vi "Dequeue Message.vi"(8 "error in (no error)":errorcluster, 10 "timeout in ms (-1)":i32=-1, 11 "Listening Queue":refnum<queue>) -> (0 "error out":errorcluster, 1 "Data":variant, 2 "Command":string, 3 "queue out":refnum<queue>, 4 "Time Stamp":timestamp, 5 "Destination":string, 7 "Source":string)   [LabVIEW 2018, in "Dynamic Reentrant.lvlib"]
uses:
  <userlib>/Dynamic Reentrant/Dynamic Reentrant.lvlib
  <userlib>/Dynamic Reentrant/Type Defs/Message.ctl
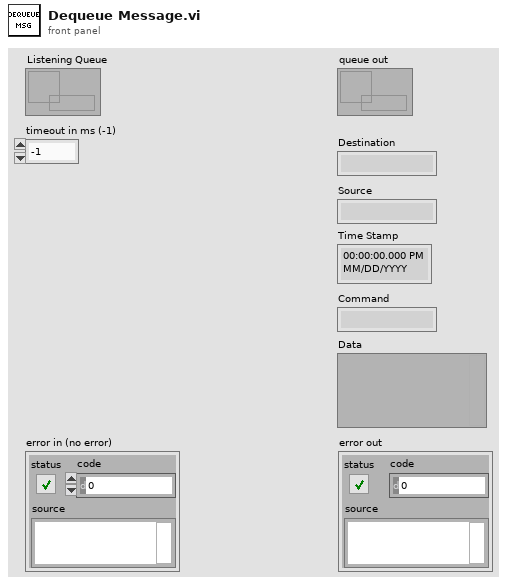
[diagram p1: front panel]
types:
  T1 = typedef "Dynamic Reentrant.lvlib/Message.ctl" = cluster{"Source":string, "Destination":string, "Time Stamp":timestamp, "Command":string, "Data":variant}
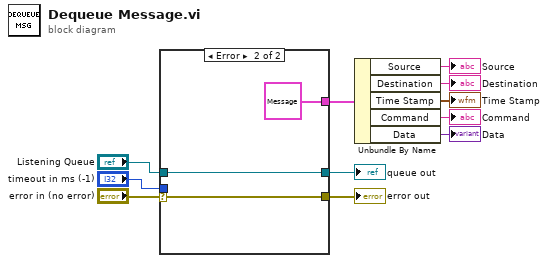
[diagram p0: block diagram]
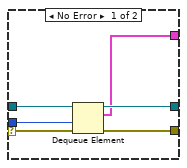
[diagram p2: hidden frame]
diagram:
  n1 = case shown="Error" "error in (no error)" {
    selector: "error in (no error)" -> [w12 w19]
    tunnel: "Listening Queue" -> [w17 w20]
    tunnel: "timeout in ms (-1)" -> [w16 _]
    tunnel: [w15 w19] -> w9
    tunnel: [w14 w20] -> w8
    tunnel: [w13 T1 {"Source"="", "Destination"="", "Time Stamp"=timestamp(0 s since 1904-01-01), "Command"="", "Data"=variant}] -> w7
    frame No Error {
      n2 = Dequeue Element(queue=w17, timeout in ms (-1)=w16, error in (no error)=w12) -> (queue out=w14:refnum<queue>, element=w13:T1, error out=w15:errorcluster)  [unwired: 1 out]
    }
    frame Error {
    }
  }
  "error out" <- w9
  "queue out" <- w8
  n3 = Unbundle By Name(w7) -> ("Source"=→"Source":string, "Destination"=→"Destination":string, "Time Stamp"=→"Time Stamp":timestamp, "Command"=→"Command":string, "Data"=→"Data":variant)
